vi "PingPong.IncWriteAddr.vi"(6 "Reset":bool, 8 "INC?":bool, 10 "End of Line":bool) -> (0 "Input Valid":bool, 3 "count":u16)   [LabVIEW 2014]
doc: "This counter counts from 0....Rollover and then returns to zero\ne.g., If rollover is 2, counter moves as 0,1,2,0,1,2.....\n\n<Latency> = 1 Tick from Reset"
panel:
  # "Copyright 2014 Vidrio Technologies\nScanImage 5 software is licensed under the Apache License, Version 2.0 (the \"License\"); you may not use any files contained\nwithin the ScanImage 5 release except in compliance with the License. You may obtain a copy of the License at\n http://www.apache.org/licenses/LICENSE-2.0\nUnless required by applicable law or agreed to in writing, software distributed under the License is distributed on an\n\"AS IS\" BASIS, WITHOUT WARRANTIES OR CONDITIONS OF ANY KIND, either express or implied. See the License for the\n specific language governing permissions and limitations under the License."
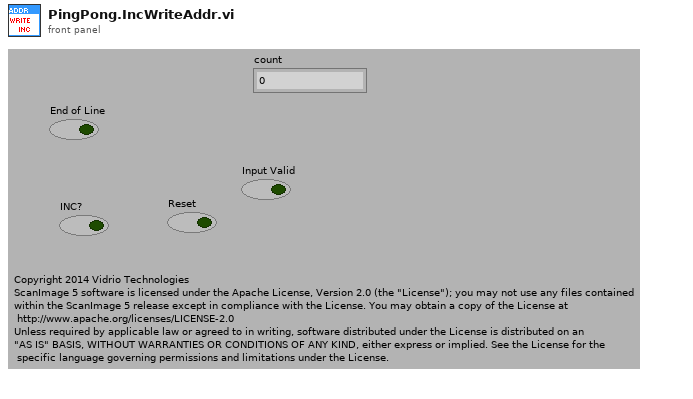
[diagram p1: front panel]
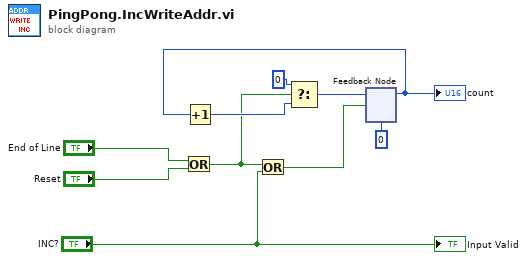
[diagram p0: block diagram]
diagram:
  n1 = Or(x="End of Line", y="Reset") -> (x .or. y?=w1:bool)
  n2 = Or(x=w1, y="INC?") -> (x .or. y?=w4:bool)
  n3 = feedback #1(u16 0) -> (w6:u16)
  "count" <- w6
  n4 = Increment(x=w6) -> (x+1=w7:u16)
  n5 = Select(t=u16 0, s=w1, f=w7) -> (s? t:f=w8:u16)
  n6 = feedback-in #1(w8, w4) -> ()
  "Input Valid" <- "INC?"
